vi "CoriFlowMessageLoop.vi"(8 "Error In":errorcluster, 11 "CommunicationRefs":T1) -> (0 "Error Out":errorcluster)   [LabVIEW 2015]
uses:
  TypeDefs/CommunicationRefs.ctl
  TypeDefs/MessageCluster.ctl
  TypeDefs/CoriFlowSettings.ctl
  TypeDefs/FluidData.ctl
  TypeDefs/FlowData.ctl
  TypeDefs/SetFlow.ctl
  <instrlib>/Bronkhorst FLOW-BUS/Public/Configure/Setpoint/Configure Setpoint (Percentage).vi
  <instrlib>/Bronkhorst FLOW-BUS/Public/Configure/Setpoint/Configure Setpoint (Direct).vi
  <instrlib>/Bronkhorst FLOW-BUS/Bronkhorst FLOW-BUS.lvlib
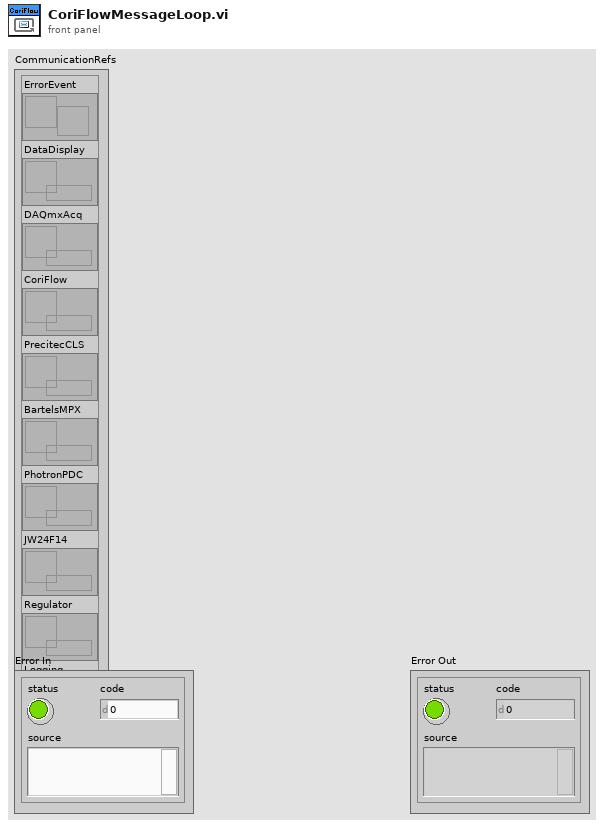
[diagram p1: front panel]
types:
  T1 = typedef "CommunicationRefs.ctl" = cluster{"ErrorEvent":refnum<user-event>, "DataDisplay":refnum<queue>, "DAQmxAcq":refnum<queue>, "CoriFlow":refnum<queue>, "PrecitecCLS":refnum<queue>, "BartelsMPX":refnum<queue>, "PhotronPDC":refnum<queue>, "JW24F14":refnum<queue>, "Regulator":refnum<queue>, "Logging":refnum<queue>}
  T2 = typedef "FluidData.ctl" = cluster{"Capacity":sgl, "Capacity Unit":string}
  T3 = typedef "FlowData.ctl" = cluster{"Setpoint Direct":sgl, "Setpoint Percentage":dbl, "Flow Direct":sgl, "Flow Percentage [%]":dbl, "Fluid Temperature [°C]":sgl, "Fluid Density [kg/m³]":sgl, "Alarm":string}
  T4 = typedef "SetFlow.ctl" = cluster{"Set Flow Value":dbl, "Set Flow Type":enum16{"Percentage", "Direct"}, "Reset Alarm":bool}
  T5 = typedef "CoriFlowSettings.ctl" = cluster{"FlowBUS COM-Port":refnum<visa-resource-name>, "Node":u8, "Baud Rate":u32, "Control Mode (0: BUS/RS232)":enum32{"BUS/RS232", "Analog input", "FLOW-BUS slave", "Valve close", "Controller idle", "Testing mode", "Tuning mode", "Setpoint 100%", "Valve fully open", "Calibration mode", "Analog slave", "Keyboard or FLOW-BUS setpoint", "Setpoint 0%", "FLOW-BUS analog slave", "(FPP) Range select mode", "(FPP) Manual start sensor select, automatic end sensor", "(FPP) Automatic start sensor select, manual end sensor", "(FPP) Automatic start and end sensor", "RS232 Setpoint", "RS232 broadcast mode", "Valve stearing (valve = setpoint)", "Analog valve stearing (valve = analog setpoint)", "Valve safe state"}, "Simulate":bool}
  T6 = enum32{"BUS/RS232", "Analog input", "FLOW-BUS slave", "Valve close", "Controller idle", "Testing mode", "Tuning mode", "Setpoint 100%", "Valve fully open", "Calibration mode", "Analog slave", "Keyboard or FLOW-BUS setpoint", "Setpoint 0%", "FLOW-BUS analog slave", "(FPP) Range select mode", "(FPP) Manual start sensor select, automatic end sensor", "(FPP) Automatic start sensor select, manual end sensor", "(FPP) Automatic start and end sensor", "RS232 Setpoint", "RS232 broadcast mode", "Valve stearing (valve = setpoint)", "Analog valve stearing (valve = analog setpoint)", "Valve safe state"}
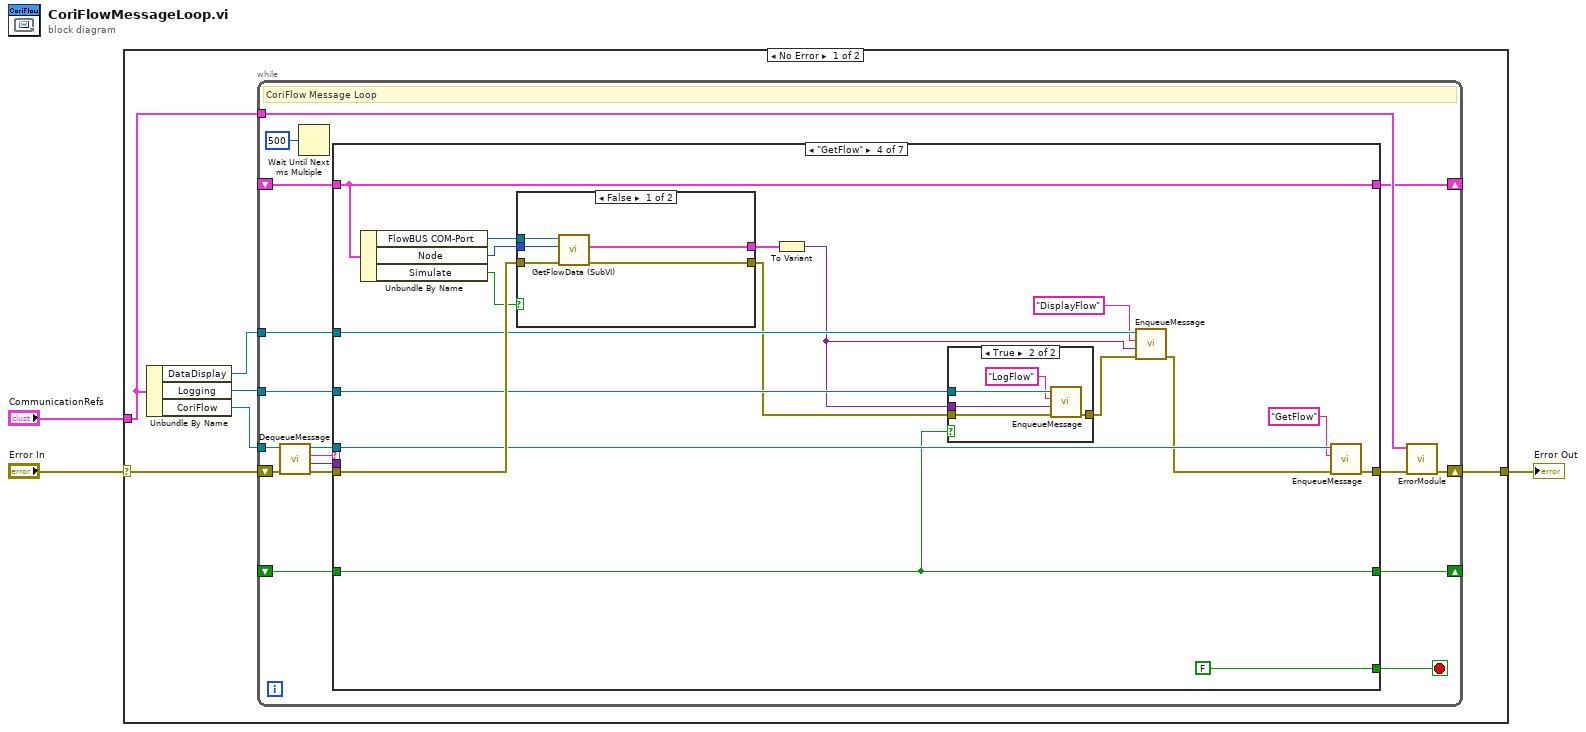
[diagram p0: block diagram]
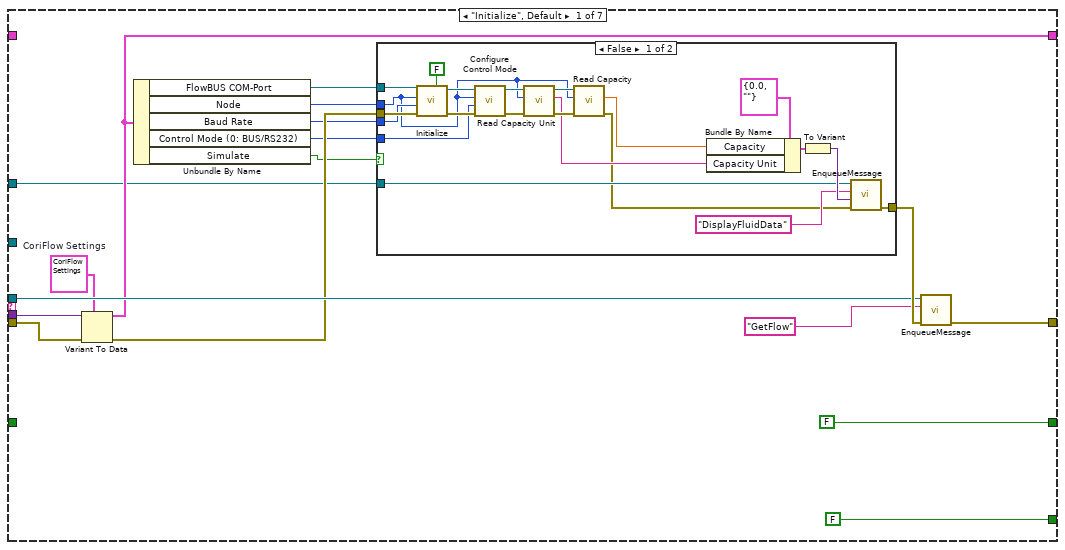
[diagram p2: hidden frame]
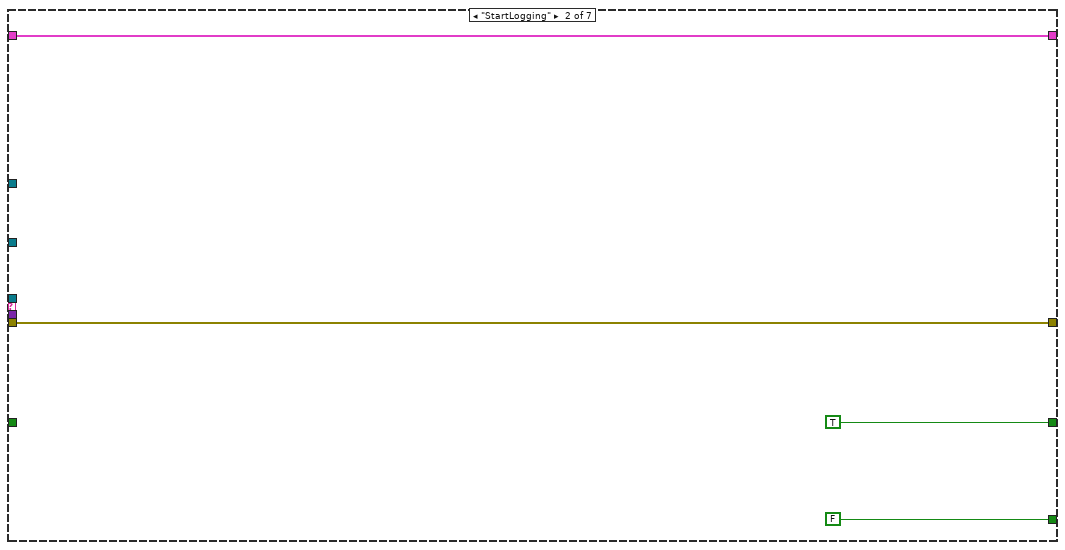
[diagram p4: hidden frame]
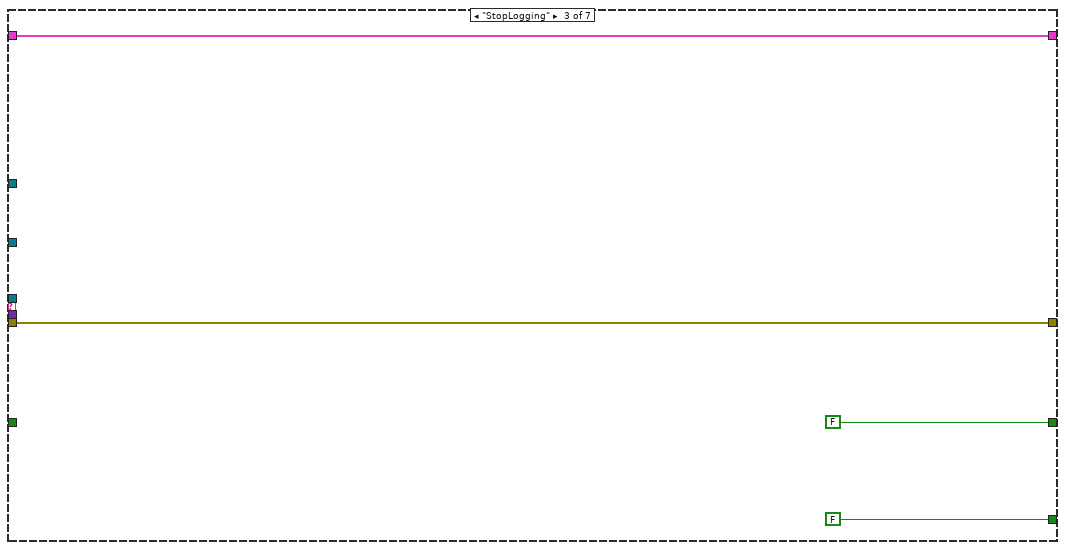
[diagram p5: hidden frame]
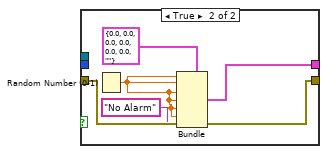
[diagram p6: hidden frame]
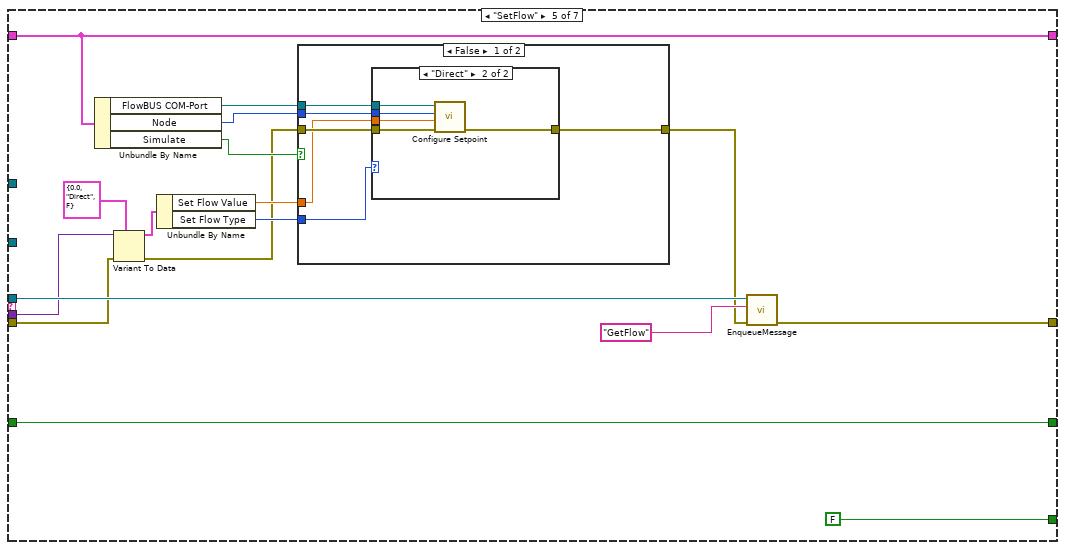
[diagram p8: hidden frame]
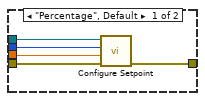
[diagram p9: hidden frame]
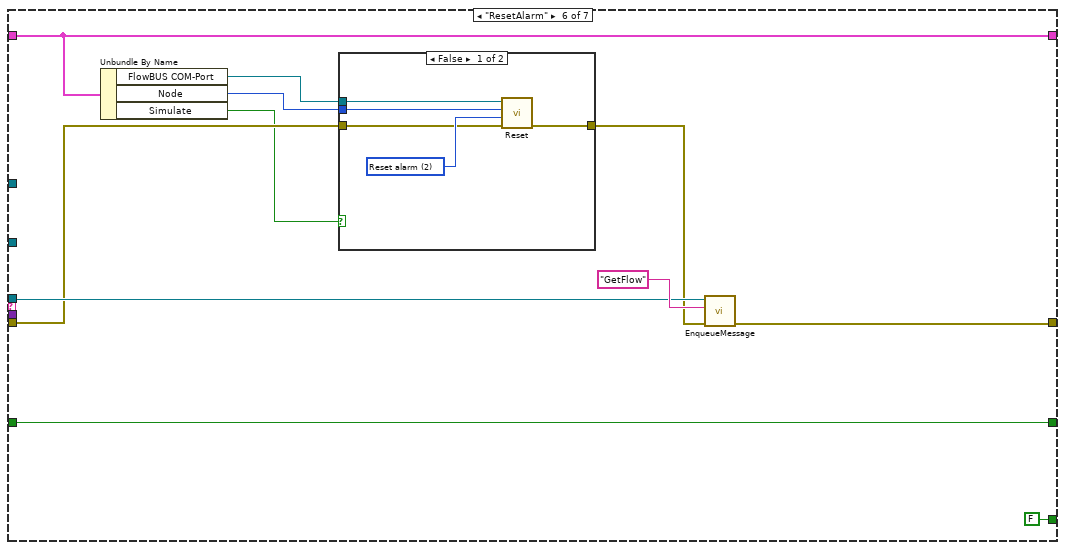
[diagram p11: hidden frame]
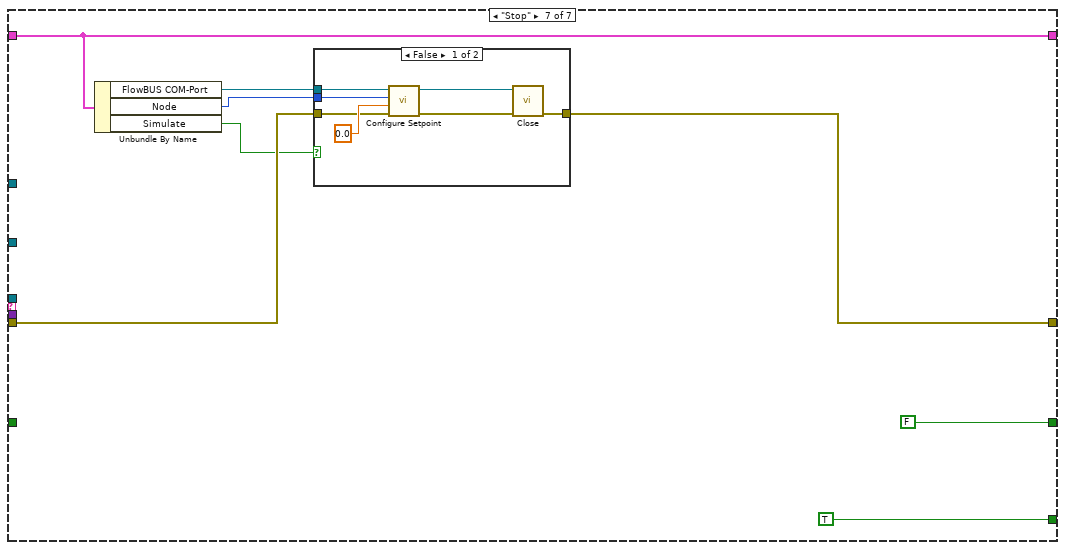
[diagram p13: hidden frame]
diagram:
  n1 = case shown="No Error" "Error In" {
    selector: "Error In" -> [w9 w175]
    tunnel: [w8 w175] -> w1
    tunnel: "CommunicationRefs" -> [w7 _]
    frame No Error {
      n2 = Unbundle By Name(w7) -> ("DataDisplay"=w5:refnum<queue>, "Logging"=w4:refnum<queue>, "CoriFlow"=w6:refnum<queue>)
      n3 = while {
        tunnel: w7 -> [w19]
        shift-right: [w21] -> w8
        shift-left: w9 -> [w26]
        tunnel: w6 -> [w16]
        shift-right: [w15] -> _
        shift-left: _ -> [w14]
        tunnel: w4 -> [w13]
        tunnel: w5 -> [w12]
        shift-right: [w11] -> _
        shift-left: _ -> [w10]
        stop <- w18 stop-if-true
        # "CoriFlow Message Loop"
        n4 = call "DequeueMessage.vi"("error in (no error)"=w26, "MessageQueue"=w16) -> ("error out"=w22:errorcluster, "MessageData"=w23:variant, "Message"=w24:string, "dupMessageQueue"=w25:refnum<queue>)  [unwired: 6 in]
        n5 = Wait Until Next ms Multiple(millisecond multiple=u32 500) -> ()  [unwired: 1 out]
        n6 = case shown="\"GetFlow\"" w24 {
          tunnel: w25 -> [w41 _ _ w87 w124 w148 _]
          tunnel: w23 -> [w36 _ _ _ w122 _ _]
          tunnel: w22 -> [w37 w67 w71 w91 w109 w145 w165]
          tunnel: [w39 w67 w71 w85 w119 w151 w164] -> w20
          tunnel: [FALSE FALSE FALSE FALSE FALSE FALSE TRUE] -> w18
          tunnel: [FALSE TRUE FALSE w82 w118 w150 FALSE] -> w15
          tunnel: w14 -> [_ _ _ w82 w118 w150 _]
          tunnel: w13 -> [_ _ _ w90 _ _ _]
          tunnel: w12 -> [w27 _ _ w89 _ _ _]
          tunnel: [w33 w66 w70 w81 w117 w147 w163] -> w11
          tunnel: w10 -> [_ w66 w70 w81 w117 w147 w163]
          frame "Initialize", Default {
            w34 = T5 {"FlowBUS COM-Port"="COM3", "Node"=1, "Baud Rate"=38400, "Control Mode (0: BUS/RS232)"=enum."BUS/RS232", "Simulate"=FALSE}  # CoriFlow Settings
            n7 = Variant To Data(error in=w37, type=w34, Variant=w36) -> (data=w33:T5, error out=w35:errorcluster)
            n8 = Unbundle By Name(w33) -> ("FlowBUS COM-Port"=w32:refnum<visa-resource-name>, "Node"=w29:u8, "Baud Rate"=w31:u32, "Control Mode (0: BUS/RS232)"=w30:T6, "Simulate"=w28:bool)
            n9 = case shown="False" w28 {
              tunnel: w35 -> [w62 w65]
              tunnel: w32 -> [w61 _]
              tunnel: w31 -> [w60 _]
              tunnel: w30 -> [w59 _]
              tunnel: w29 -> [w53 _]
              tunnel: w27 -> [w49 _]
              tunnel: [w45 w65] -> w43
              frame False {
                n10 = call <instrlib>:"Initialize.vi"("Reset (False)"=FALSE, "error in (no error)"=w62, "Baud Rate (38400)"=w60, "Node (3)"=w53, "VISA resource name"=w61) -> ("error out"=w63:errorcluster, "VISA resource name out"=w58:refnum<visa-resource-name>)  [unwired: 5 in]
                n11 = call <instrlib>:"Configure Control Mode.vi"("error in (no error)"=w63, "Control Mode (0: BUS/RS232)"=w59, "Node (3)"=w53, "VISA resource name"=w58) -> ("error out"=w57:errorcluster, "VISA resource name out"=w56:refnum<visa-resource-name>)  [unwired: 6 in]
                n12 = call <instrlib>:"Read Capacity Unit.vi"("error in (no error)"=w57, "Node (3)"=w53, "VISA resource name"=w56) -> ("error out"=w55:errorcluster, "Capacity Unit"=w47:string, "VISA resource name out"=w54:refnum<visa-resource-name>)  [unwired: 6 in]
                n13 = call <instrlib>:"Read Capacity.vi"("error in (no error)"=w55, "Node (3)"=w53, "VISA resource name"=w54) -> ("error out"=w44:errorcluster, "Capacity"=w48:sgl)  [unwired: 6 in, 1 out]
                n14 = Bundle By Name(cluster=T2 {"Capacity"=0.0, "Capacity Unit"=""} ("Fluid Data"), "Capacity"=w48, "Capacity Unit"=w47) -> (w51:T2)
                n15 = To Variant(anything=w51) -> (Variant=w50:variant)
                n16 = call "EnqueueMessage.vi"("error in (no error)"=w44, "MessageData"=w50, "Message"="DisplayFluidData", "MessageQueue"=w49) -> ("error out"=w45:errorcluster)  [unwired: 6 in, 1 out]
              }
              frame True {
              }
            }
            n17 = call "EnqueueMessage.vi"("error in (no error)"=w43, "Message"="GetFlow", "MessageQueue"=w41) -> ("error out"=w39:errorcluster)  [unwired: 7 in, 1 out]
          }
          frame "StartLogging" {
          }
          frame "StopLogging" {
          }
          frame "GetFlow" {
            n18 = Unbundle By Name(w81) -> ("FlowBUS COM-Port"=w80:refnum<visa-resource-name>, "Node"=w79:u8, "Simulate"=w78:bool)
            n19 = case shown="False" w78 {
              tunnel: w91 -> [w96 w99]
              tunnel: w80 -> [w95 _]
              tunnel: w79 -> [w94 _]
              tunnel: [w93 w100] -> w76
              tunnel: [w92 w99] -> w75
              frame False {
                n20 = call "GetFlowData (SubVI).vi"("error in (no error)"=w96, "Node"=w94, "VISA Refnum in"=w95) -> ("error out"=w92:errorcluster, "Flow Data"=w93:T3)  [unwired: 6 in]
              }
              frame True {
                n21 = Random Number (0-1)() -> (number: 0 to 1=w97:dbl)
                n22 = Bundle(cluster=T3 {"Setpoint Direct"=0.0, "Setpoint Percentage"=0.0, "Flow Direct"=0.0, "Flow Percentage [%]"=0.0, "Fluid Temperature [°C]"=0.0, "Fluid Density [kg/m³]"=0.0, "Alarm"=""} ("Sensor Data"), "Setpoint Direct"=w97, "Setpoint Percentage"=w97, "Flow Direct"=w97, "Flow Percentage [%]"=w97, "Fluid Temperature [°C]"=w97, "Fluid Density [kg/m³]"=w97, "Alarm"="No Alarm") -> (w100:T3)
              }
            }
            n23 = To Variant(anything=w76) -> (Variant=w77:variant)
            n24 = case shown="True" w82 {
              tunnel: w90 -> [_ w107]
              tunnel: [w102 w105] -> w83
              tunnel: w77 -> [_ w104]
              tunnel: w75 -> [w102 w103]
              frame False {
              }
              frame True {
                n25 = call "EnqueueMessage.vi"("error in (no error)"=w103, "MessageData"=w104, "Message"="LogFlow", "MessageQueue"=w107) -> ("error out"=w105:errorcluster)  [unwired: 6 in, 1 out]
              }
            }
            n26 = call "EnqueueMessage.vi"("error in (no error)"=w83, "MessageData"=w77, "Message"="DisplayFlow", "MessageQueue"=w89) -> ("error out"=w74:errorcluster)  [unwired: 6 in, 1 out]
            n27 = call "EnqueueMessage.vi"("error in (no error)"=w74, "Message"="GetFlow", "MessageQueue"=w87) -> ("error out"=w85:errorcluster)  [unwired: 7 in, 1 out]
          }
          frame "SetFlow" {
            n28 = Unbundle By Name(w117) -> ("FlowBUS COM-Port"=w116:refnum<visa-resource-name>, "Node"=w115:u8, "Simulate"=w114:bool)
            n29 = Variant To Data(error in=w109, type=T4 {"Set Flow Value"=0.0, "Set Flow Type"=enum."Direct", "Reset Alarm"=FALSE} ("Set Flow"), Variant=w122) -> (data=w112:T4, error out=w108:errorcluster)
            n30 = Unbundle By Name(w112) -> ("Set Flow Value"=w111:dbl, "Set Flow Type"=w110:enum16{"Percentage", "Direct"})
            n31 = case shown="False" w114 {
              tunnel: w108 -> [w130 w141]
              tunnel: [w129 w141] -> w120
              tunnel: w116 -> [w128 _]
              tunnel: w115 -> [w127 _]
              tunnel: w111 -> [w126 _]
              tunnel: w110 -> [w125 _]
              frame False {
                n32 = case shown="\"Direct\"" w125 {
                  tunnel: w130 -> [w135 w138]
                  tunnel: [w134 w139] -> w129
                  tunnel: w128 -> [w133 w140]
                  tunnel: w127 -> [w132 w137]
                  tunnel: w126 -> [w131 w136]
                  frame "Percentage", Default {
                    n33 = call-poly <instrlib>:"Configure Setpoint.vi"("error in (no error)"=w135, "Setpoint Percentage (0%)"=w131, "Node (3)"=w132, "VISA resource name"=w133) -> ("error out"=w134:errorcluster)  [unwired: 6 in, 1 out]
                  }
                  frame "Direct" {
                    n34 = call-poly <instrlib>:"Configure Setpoint.vi"("error in (no error)"=w138, "Setpoint Direct (0)"=w136, "Node (3)"=w137, "VISA resource name"=w140) -> ("error out"=w139:errorcluster)  [unwired: 6 in, 1 out]
                  }
                }
              }
              frame True {
              }
            }
            n35 = call "EnqueueMessage.vi"("error in (no error)"=w120, "Message"="GetFlow", "MessageQueue"=w124) -> ("error out"=w119:errorcluster)  [unwired: 7 in, 1 out]
          }
          frame "ResetAlarm" {
            n36 = Unbundle By Name(w147) -> ("FlowBUS COM-Port"=w146:refnum<visa-resource-name>, "Node"=w144:u8, "Simulate"=w142:bool)
            n37 = case shown="False" w142 {
              tunnel: w146 -> [w156 _]
              tunnel: w145 -> [w155 w158]
              tunnel: w144 -> [w154 _]
              tunnel: [w153 w158] -> w143
              frame False {
                w157 = u32 2 items=["No Reset", "Reset counter value (no mode change)", "Reset alarm", "Restart batch counter", "Reset counter value (counter off)", "Soft Reset"] ("Reset mode (5: Soft Reset)")
                n38 = call <instrlib>:"Reset.vi"("error in (no error)"=w155, "Reset mode (5: Soft Reset)"=w157, "Node (3)"=w154, "VISA resource name"=w156) -> ("error out"=w153:errorcluster)  [unwired: 6 in, 1 out]
              }
              frame True {
              }
            }
            n39 = call "EnqueueMessage.vi"("error in (no error)"=w143, "Message"="GetFlow", "MessageQueue"=w148) -> ("error out"=w151:errorcluster)  [unwired: 7 in, 1 out]
          }
          frame "Stop" {
            n40 = Unbundle By Name(w163) -> ("FlowBUS COM-Port"=w162:refnum<visa-resource-name>, "Node"=w161:u8, "Simulate"=w160:bool)
            n41 = case shown="False" w160 {
              tunnel: w165 -> [w172 w174]
              tunnel: [w168 w174] -> w164
              tunnel: w162 -> [w171 _]
              tunnel: w161 -> [w170 _]
              frame False {
                n42 = call-poly <instrlib>:"Configure Setpoint.vi"("error in (no error)"=w172, "Setpoint Percentage (0%)"=0.0, "Node (3)"=w170, "VISA resource name"=w171) -> ("error out"=w169:errorcluster, "VISA resource name out"=w167:refnum<visa-resource-name>)  [unwired: 6 in]
                n43 = call <instrlib>:"Close.vi"("error in (no error)"=w169, "VISA resource name"=w167) -> ("error out"=w168:errorcluster)  [unwired: 9 in]
              }
              frame True {
              }
            }
          }
        }
        n44 = call "ErrorModule.vi"("Error In"=w20, "CommunicationRefs"=w19) -> ("Error Out"=w21:errorcluster)  [unwired: 9 in]
      }
    }
    frame Error {
    }
  }
  "Error Out" <- w1
